vi "toml_value_datetime_parse.vi"(8 "error in (no error)":errorcluster, 11 "toml":string) -> (0 "error out":errorcluster, 3 "time stamp":timestamp format="%<%H:%M:%S%6u\n%Y/%m/%d>T")   [LabVIEW 2017]
uses:
  <vilib>/Utility/miscctls.llb/LVDateTimeRec.ctl
  <vilib>/regexp/Match Regular Expression.xnode
panel:
  out "date time":T1
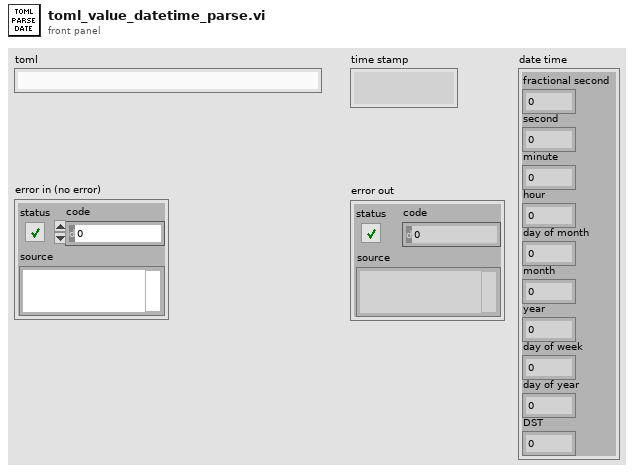
[diagram p1: front panel]
types:
  T1 = typedef "LVDateTimeRec.ctl" = cluster{"fractional second":dbl, "second":i32, "minute":i32, "hour":i32, "day of month":i32, "month":i32, "year":i32, "day of week":i32, "day of year":i32, "DST":i32}
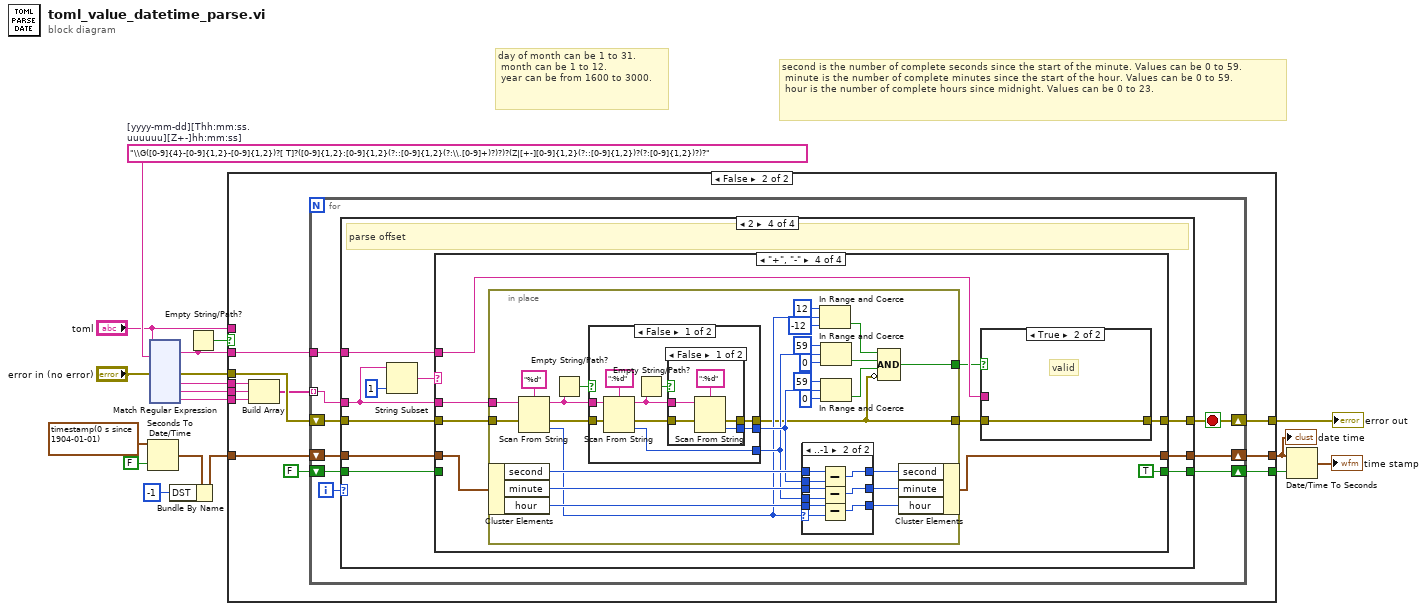
[diagram p0: block diagram]
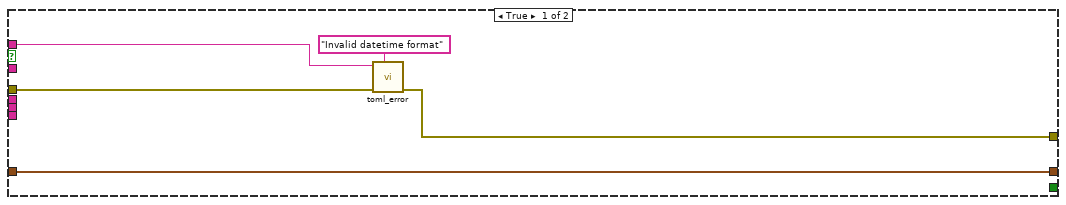
[diagram p2: hidden frame]
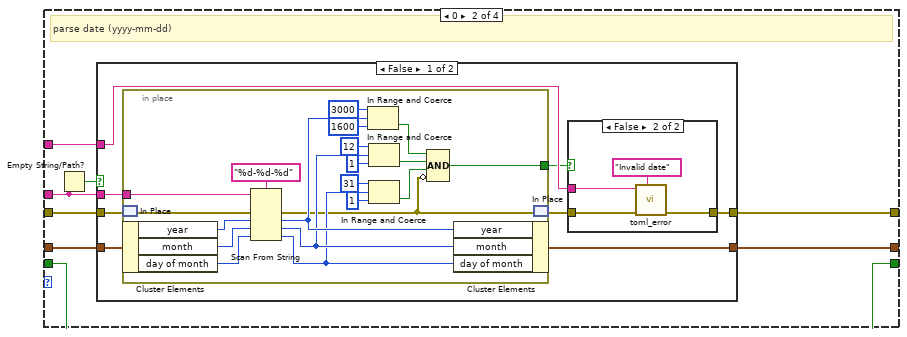
[diagram p4: hidden frame]
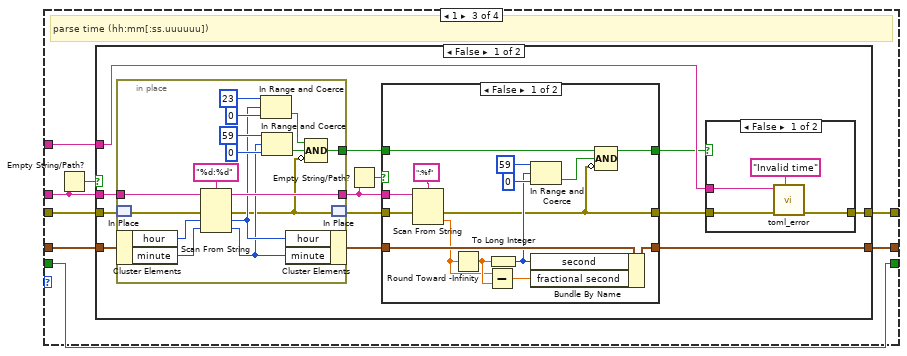
[diagram p7: hidden frame]
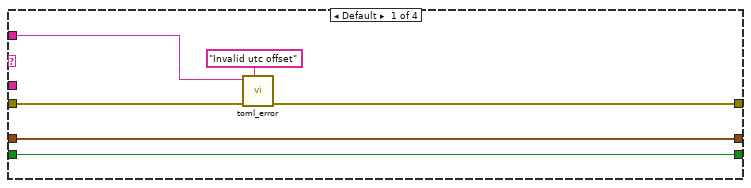
[diagram p11: hidden frame]
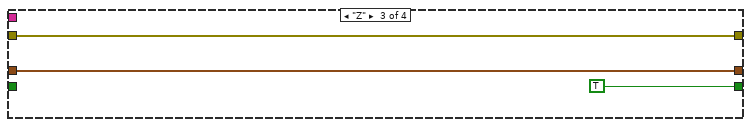
[diagram p13: hidden frame]
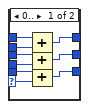
[diagram p14: hidden frame]
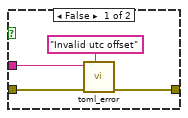
[diagram p17: hidden frame]
diagram:
  w18 = "\\G([0-9]{4}-[0-9]{1,2}-[0-9]{1,2})?[ T]?([0-9]{1,2}:[0-9]{1,2}(?::[0-9]{1,2}(?:\\.[0-9]+)?)?)?(Z|[+-][0-9]{1,2}(?::[0-9]{1,2})?(?:[0-9]{1,2})?)?"  # [yyyy-mm-dd][Thh:mm:ss.uuuuuu][Z+-]hh:mm:ss]
  # "second is the number of complete seconds since the start of the minute. Values can be 0 to 59.  \n minute is the number of complete minutes since the start of the hour. Values can be 0 to 59.  \n hour is the number of complete hours since midnight. Values can be 0 to 23."
  # "day of month can be 1 to 31.  \n month can be 1 to 12.  \n year can be from 1600 to 3000."
  n1 = Seconds To Date/Time(time stamp (now)=timestamp(0 s since 1904-01-01) ("time stamp"), to UTC (F)=FALSE) -> (date time rec=w2:T1)
  n2 = xnode "Match Regular Expression"("input string"="toml", "regular expression"=w18, "error in"="error in (no error)") -> ("whole match"=w10:string, "error out"=w17:errorcluster, "submatch 1"=w14:string, "submatch 2"=w16:string, "submatch 3"=w15:string)  [unwired: 3 in, 3 out]
  n3 = Bundle By Name(cluster=w2, "DST"=-1) -> (w1:T1)
  n4 = Empty String/Path?(string/path=w10) -> (empty?=w9:bool)
  n5 = case shown="False" w9 {
    tunnel: w17 -> [w22 w34]
    tunnel: w10 -> [_ w33]
    tunnel: w16 -> [_ w32]
    tunnel: w15 -> [_ w31]
    tunnel: w14 -> [_ w30]
    tunnel: [w20 w28] -> w12
    tunnel: "toml" -> [w21 _]
    tunnel: w1 -> [w19 w26]
    tunnel: [_ w25] -> w6
    tunnel: [w19 w24] -> w5
    frame True {
      n6 = call "toml_error.vi"("message"="Invalid datetime format", "error in (no error)"=w22, "toml"=w21) -> ("error out"=w20:errorcluster)  [unwired: 8 in]
    }
    frame False {
      n7 = Build Array(w30, w32, w31) -> (w29:string[])
      n8 = for {
        tunnel: w33 -> [w41]
        tunnel: w29 -> [w40] mode=indexing
        shift-right: [w39] -> w24
        shift-left: w26 -> [w42]
        shift-right: [w37] -> w28
        shift-left: w34 -> [w43]
        shift-right: [w36] -> w25
        shift-left: FALSE -> [w35]
        i -> [w38]
        stop <- w37 stop-if-true
        n9 = case shown="2" w38 {
          tunnel: w43 -> [w45 w54 w97 w160]
          tunnel: w42 -> [w46 w53 w96 w158]
          tunnel: w41 -> [_ w51 w94 w157]
          tunnel: w40 -> [_ w50 w93 w156]
          tunnel: [w46 w49 w92 w159] -> w39
          tunnel: [w45 w48 w91 w161] -> w37
          tunnel: [w44 w47 w90 w153] -> w36
          tunnel: w35 -> [w44 w47 w90 w152]
          frame Default {
          }
          frame 0 {
            # "parse date (yyyy-mm-dd)"
            n10 = Empty String/Path?(string/path=w50) -> (empty?=w52:bool)
            n11 = case shown="False" w52 {
              tunnel: w50 -> [w62 _]
              tunnel: w54 -> [w60 w88]
              tunnel: w53 -> [w61 w89]
              tunnel: w51 -> [w56 _]
              tunnel: [w59 w88] -> w48
              tunnel: [w58 w89] -> w49
              frame False {
                n12 = in-place {
                  in-place-border: w62 -> [w87]
                  in-place-border: [w68] -> w55
                  n13 = in-place-match #1(w60) -> (w82:errorcluster)
                  n14 = in-place-cluster #2(w61) -> ("year"=w85:i32, "month"=w84:i32, "day of month"=w83:i32)
                  n15 = Scan From String(format string="%d-%d-%d", input string=w87, error in=w82, default 1=w85, default 2=w84, default 3=w83) -> (error out=w69:errorcluster, output 1=w81:i32, output 2=w75:i32, output 3=w70:i32)  [unwired: 1 in, 2 out]
                  n16 = In Range and Coerce(upper limit=3000, x=w81, lower limit=1600) -> (In Range?=w78:bool)  [unwired: 1 out]
                  n17 = In Range and Coerce(upper limit=12, x=w75, lower limit=1) -> (In Range?=w74:bool)  [unwired: 1 out]
                  n18 = In Range and Coerce(upper limit=31, x=w70, lower limit=1) -> (In Range?=w71:bool)  [unwired: 1 out]
                  n19 = Compound Arithmetic op=AND(w78, w74, w71, invert w69) -> (w68:bool)
                  n20 = in-place-cluster #2("year"=w81, "month"=w75, "day of month"=w70) -> (w58:T1)
                  n21 = in-place-match #1(w69) -> (w57:errorcluster)
                }
                n22 = case shown="False" w55 {
                  tunnel: w56 -> [_ w67]
                  tunnel: [w63 w65] -> w59
                  tunnel: w57 -> [w63 w64]
                  frame True {
                    # "valid date"
                  }
                  frame False {
                    n23 = call "toml_error.vi"("message"="Invalid date", "error in (no error)"=w64, "toml"=w67) -> ("error out"=w65:errorcluster)  [unwired: 8 in]
                  }
                }
              }
              frame True {
              }
            }
          }
          frame 1 {
            # "parse time (hh:mm[:ss.uuuuuu])"
            n24 = Empty String/Path?(string/path=w93) -> (empty?=w95:bool)
            n25 = case shown="False" w95 {
              tunnel: w93 -> [w110 _]
              tunnel: w97 -> [w108 w151]
              tunnel: w96 -> [w109 w150]
              tunnel: w94 -> [w100 _]
              tunnel: [w107 w151] -> w91
              tunnel: [w103 w150] -> w92
              frame False {
                n26 = in-place {
                  in-place-border: w110 -> [w149]
                  in-place-border: [w144] -> w102
                  in-place-border: [w135] -> w99
                  n27 = in-place-match #3(w108) -> (w145:errorcluster)
                  n28 = in-place-cluster #4(w109) -> ("hour"=w147:i32, "minute"=w146:i32)
                  n29 = Scan From String(format string="%d:%d", input string=w149, error in=w145, default 1=w147, default 2=w146) -> (remaining string=w144:string, error out=w134:errorcluster, output 1=w138:i32, output 2=w136:i32)  [unwired: 1 in, 1 out]
                  n30 = In Range and Coerce(upper limit=23, x=w138, lower limit=0) -> (In Range?=w142:bool)  [unwired: 1 out]
                  n31 = In Range and Coerce(upper limit=59, x=w136, lower limit=0) -> (In Range?=w139:bool)  [unwired: 1 out]
                  n32 = in-place-cluster #4("hour"=w138, "minute"=w136) -> (w106:T1)
                  n33 = Compound Arithmetic op=AND(w142, w139, invert w134) -> (w135:bool)
                  n34 = in-place-match #3(w134) -> (w105:errorcluster)
                }
                n35 = Empty String/Path?(string/path=w102) -> (empty?=w101:bool)
                n36 = case shown="False" w101 {
                  tunnel: w106 -> [w125 w127]
                  tunnel: w105 -> [w124 w128]
                  tunnel: w102 -> [w123 _]
                  tunnel: [w112 w128] -> w104
                  tunnel: [w122 w127] -> w103
                  tunnel: w99 -> [w114 w126]
                  tunnel: [w111 w126] -> w98
                  frame False {
                    n37 = Scan From String(format string=":%f", input string=w123, error in=w124) -> (error out=w112:errorcluster, output 1=w119:dbl)  [unwired: 2 in, 2 out]
                    n38 = Round Toward -Infinity(1:w119) -> (0:w120:dbl)
                    n39 = Subtract(x=w119, y=w120) -> (x-y=w118:dbl)
                    n40 = To Long Integer(number=w120) -> (32bit integer=w115:i32)
                    n41 = In Range and Coerce(upper limit=59, x=w115, lower limit=0) -> (In Range?=w113:bool)  [unwired: 1 out]
                    n42 = Bundle By Name(cluster=w125, "second"=w115, "fractional second"=w118) -> (w122:T1)
                    n43 = Compound Arithmetic op=AND(w114, w113, invert w112) -> (w111:bool)
                  }
                  frame True {
                  }
                }
                n44 = case shown="False" w98 {
                  tunnel: w100 -> [w131 _]
                  tunnel: [w129 w133] -> w107
                  tunnel: w104 -> [w132 w133]
                  frame False {
                    n45 = call "toml_error.vi"("message"="Invalid time", "error in (no error)"=w132, "toml"=w131) -> ("error out"=w129:errorcluster)  [unwired: 8 in]
                  }
                  frame True {
                    # "valid"
                  }
                }
              }
              frame True {
              }
            }
          }
          frame 2 {
            # "parse offset"
            n46 = String Subset(string=w156, length (rest)=1 ("length (rest)")) -> (substring=w154:string)  [unwired: 1 in]
            n47 = case shown="\"+\", \"-\"" w154 {
              tunnel: [w165 w170 w173 w178] -> w161
              tunnel: w160 -> [w166 w170 w173 w182]
              tunnel: [w163 w169 w172 w175] -> w159
              tunnel: w158 -> [w163 w169 w172 w176]
              tunnel: w157 -> [w164 _ _ w179]
              tunnel: w156 -> [_ _ _ w181]
              tunnel: [w162 w168 TRUE TRUE] -> w153
              tunnel: w152 -> [w162 w168 _ _]
              frame Default {
                n48 = call "toml_error.vi"("message"="Invalid utc offset", "error in (no error)"=w166, "toml"=w164) -> ("error out"=w165:errorcluster)  [unwired: 8 in]
              }
              frame "" {
              }
              frame "Z" {
              }
              frame "+", "-" {
                n49 = in-place {
                  in-place-border: w182 -> [w208]
                  in-place-border: w181 -> [w207]
                  in-place-border: [w184] -> w180
                  in-place-border: [w183] -> w174
                  n50 = in-place-cluster #5(w176) -> ("second"=w201:i32, "minute"=w200:i32, "hour"=w197:i32)
                  n51 = Scan From String(format string="%d", input string=w207, error in=w208) -> (remaining string=w204:string, error out=w205:errorcluster, output 1=w186:i32)  [unwired: 2 in, 1 out]
                  n52 = Empty String/Path?(string/path=w204) -> (empty?=w203:bool)
                  n53 = case shown="False" w203 {
                    tunnel: w205 -> [w234 w242]
                    tunnel: w204 -> [w233 _]
                    tunnel: [w229 w242] -> w184
                    tunnel: [w228 _] -> w188
                    tunnel: [w227 _] -> w187
                    frame False {
                      n54 = Scan From String(format string=":%d", input string=w233, error in=w234) -> (remaining string=w230:string, error out=w231:errorcluster, output 1=w227:i32)  [unwired: 2 in, 1 out]
                      n55 = Empty String/Path?(string/path=w230) -> (empty?=w232:bool)
                      n56 = case shown="False" w232 {
                        tunnel: w231 -> [w239 w241]
                        tunnel: w230 -> [w238 _]
                        tunnel: [w237 w241] -> w229
                        tunnel: [w236 _] -> w228
                        frame False {
                          n57 = Scan From String(format string=":%d", input string=w238, error in=w239) -> (error out=w237:errorcluster, output 1=w236:i32)  [unwired: 2 in, 2 out]
                        }
                        frame True {
                        }
                      }
                    }
                    frame True {
                    }
                  }
                  n58 = case shown="..-1" w186 {
                    selector: w186 -> [w209 w218]
                    tunnel: [w214 w223] -> w202
                    tunnel: w201 -> [w217 w226]
                    tunnel: w200 -> [w216 w225]
                    tunnel: [w213 w222] -> w199
                    tunnel: [w212 w221] -> w198
                    tunnel: w197 -> [w215 w224]
                    tunnel: w188 -> [w211 w220]
                    tunnel: w187 -> [w210 w219]
                    frame 0.. {
                      n59 = Add(x=w217, y=w211) -> (x+y=w214:i32)
                      n60 = Add(x=w216, y=w210) -> (x+y=w213:i32)
                      n61 = Add(x=w215, y=w209) -> (x+y=w212:i32)
                    }
                    frame ..-1 {
                      n62 = Subtract(x=w226, y=w220) -> (x-y=w223:i32)
                      n63 = Subtract(x=w225, y=w219) -> (x-y=w222:i32)
                      n64 = Subtract(x=w224, y=w218) -> (x-y=w221:i32)
                    }
                  }
                  n65 = In Range and Coerce(upper limit=12, x=w186, lower limit=-12) -> (In Range?=w195:bool)  [unwired: 1 out]
                  n66 = In Range and Coerce(upper limit=59, x=w187, lower limit=0) -> (In Range?=w192:bool)  [unwired: 1 out]
                  n67 = In Range and Coerce(upper limit=59, x=w188, lower limit=0) -> (In Range?=w185:bool)  [unwired: 1 out]
                  n68 = Compound Arithmetic op=AND(w195, w192, w185, invert w184) -> (w183:bool)
                  n69 = in-place-cluster #5("second"=w202, "minute"=w199, "hour"=w198) -> (w175:T1)
                }
                n70 = case shown="True" w174 {
                  tunnel: w179 -> [w246 _]
                  tunnel: [w244 w247] -> w178
                  tunnel: w180 -> [w243 w247]
                  frame False {
                    n71 = call "toml_error.vi"("message"="Invalid utc offset", "error in (no error)"=w243, "toml"=w246) -> ("error out"=w244:errorcluster)  [unwired: 8 in]
                  }
                  frame True {
                    # "valid"
                  }
                }
              }
            }
          }
        }
      }
    }
  }
  "error out" <- w12
  "date time" <- w5
  n72 = Date/Time To Seconds(1:w6, 2:w5) -> (0:→"time stamp":timestamp)
